vi "Duzy wykres 1.vi"(6 "Wolna?":bool, 8 "error in (no error)":errorcluster, 10 "okno":dbl) -> (0 "error out":errorcluster)   [LabVIEW 2014]
doc: "Use this template to build a VI to use as a subVI."
uses:
  Kontrolki/FVGs/FVG akcje podstawowa.ctl
panel:
  out "Waveform Graph":waveform(dbl)[](graph)
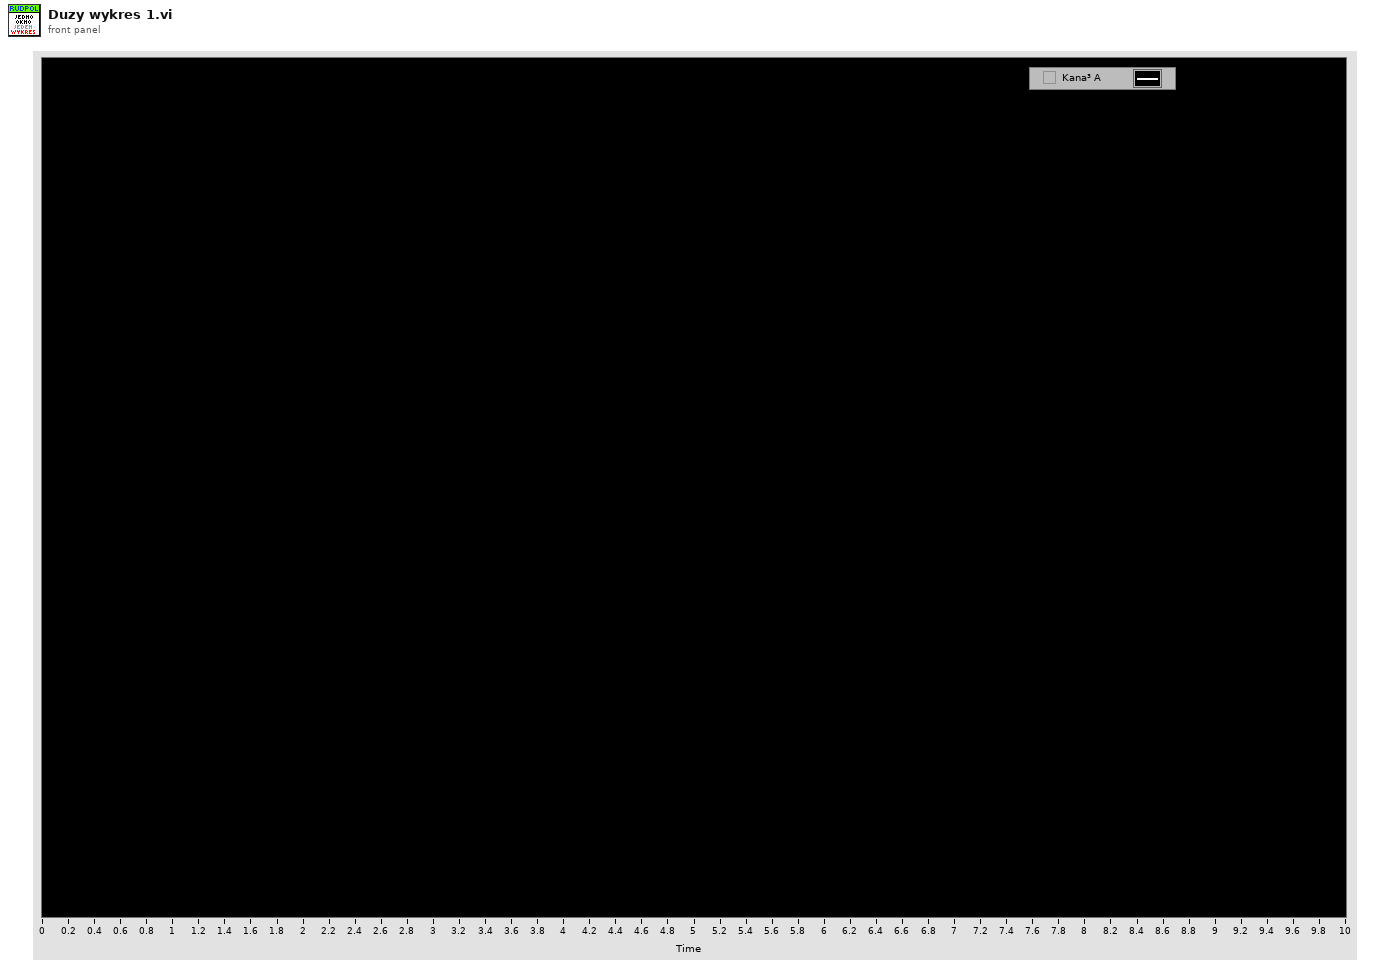
[diagram p1: front panel]
types:
  T1 = typedef "FVG akcje podstawowa.ctl" = enum16{"GET", "SET"}
  T2 = typedef "Kanaly.ctl" = cluster{"Analogowe":waveform(dbl)[], "Cyfrowe":waveform(dbl)[], "Zwarcie":waveform(dbl)[], "Enkoder":waveform(dbl)[]}
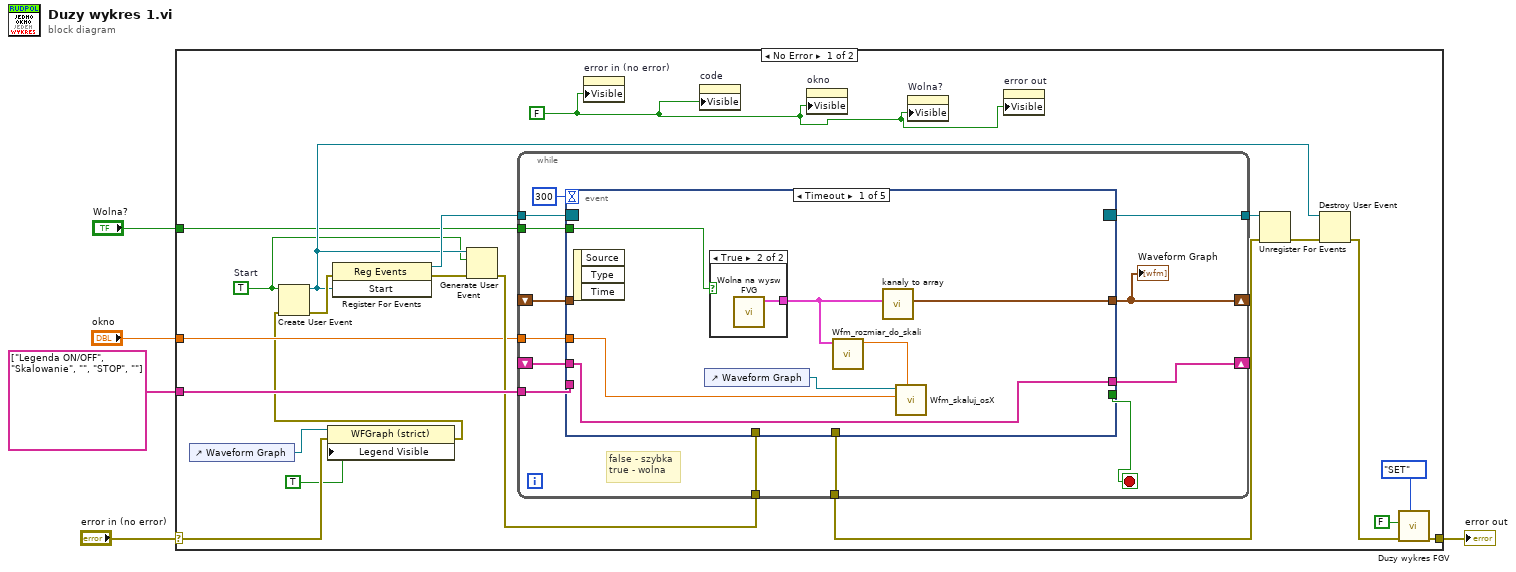
[diagram p0: block diagram]
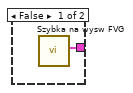
[diagram p2: hidden frame]
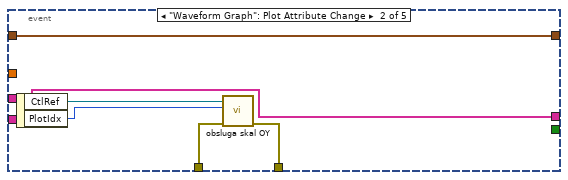
[diagram p3: hidden frame]
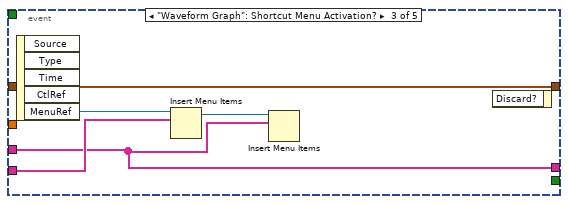
[diagram p4: hidden frame]
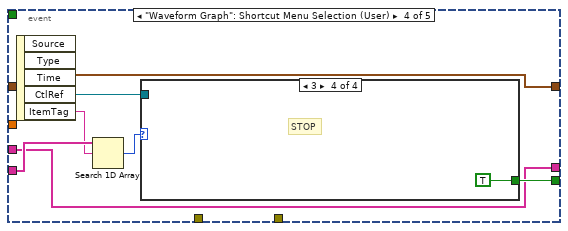
[diagram p5: hidden frame]
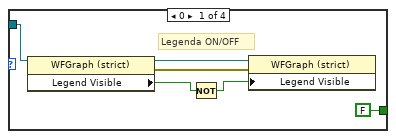
[diagram p6: hidden frame]
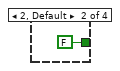
[diagram p7: hidden frame]
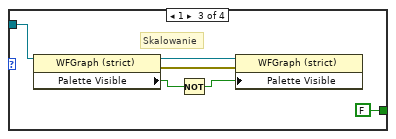
[diagram p8: hidden frame]
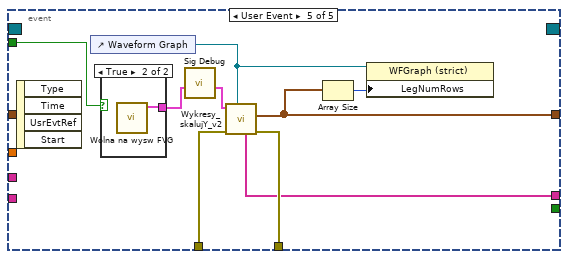
[diagram p9: hidden frame]
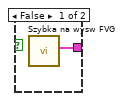
[diagram p10: hidden frame]
diagram:
  n1 = case shown="No Error" "error in (no error)" {
    selector: "error in (no error)" -> [w11 w92]
    tunnel: [w24 w92] -> w4
    tunnel: string[] ["Legenda ON/OFF", "Skalowanie", "", "STOP", ""] -> [w23 _]
    tunnel: "okno" -> [w12 _]
    tunnel: "Wolna?" -> [w7 _]
    frame No Error {
      w13 = TRUE  # Start
      w6 = FALSE ("Visible")
      n2 = control-ref of="Waveform Graph"() -> (w9:refnum<vi>)
      n3 = property class="WFGraph (strict)"(reference=w9, error in=w11, "Legend Visible"=TRUE ("Legend:Visible")) -> (error out=w10:errorcluster)  [unwired: 1 out]
      n4 = Create User Event(user event datatype=w13, error in=w10) -> (user event=w16:refnum<user-event>, error out=w21:errorcluster)
      n5 = register-events(error in=w21, w16) -> (reference out=w22:refnum<event-registration>, error out=w20:errorcluster)  [unwired: 1 in]
      n6 = Generate User Event(user event=w16, event data cluster=w13, error in=w20) -> (error out=w19:errorcluster)  [unwired: 1 in, 1 out]
      n7 = while {
        tunnel: w19 -> [w39]
        tunnel: [w38] -> w15
        tunnel: w23 -> [w36]
        tunnel: w22 -> [w34]
        tunnel: [w33] -> w18
        tunnel: w12 -> [w32]
        shift-right: [w31] -> _
        shift-left: _ -> [w30]
        tunnel: w7 -> [w29]
        shift-right: [w28] -> _
        shift-left: _ -> [w27]
        stop <- w35 stop-if-true
        # "false - szybka\ntrue - wolna"
        n8 = event shown="[0] Timeout" {
          selector: w34 -> [_ _ _ _ _]
          dyn-events: [_ _ _ _ _] -> w33
          timeout: 300 -> [_ _ _ _ _]
          tunnel: w39 -> [_ w51 _ _ w88]
          tunnel: [_ w50 _ _ w87] -> w38
          tunnel: w36 -> [_ _ w58 w66 _]
          tunnel: [_ _ _ w62 _] -> w35
          tunnel: [w46 w52 w57 w61 w86] -> w31
          tunnel: w32 -> [w42 _ _ _ _]
          tunnel: w30 -> [_ w52 w57 w61 _]
          tunnel: w29 -> [w41 _ _ _ w84]
          tunnel: [w40 w49 w56 w60 w81] -> w28
          tunnel: w27 -> [w40 w49 w56 w60 _]
          event Timeout {
            n9 = event-data() -> ()  [unwired: 1 in, 3 out]
            n10 = control-ref of="Waveform Graph"() -> (w43:refnum<vi>)
            n11 = case shown="True" w41 {
              tunnel: [w47 w48] -> w45
              frame False {
                n12 = call "Szybka na wysw FVG.vi"() -> ("Bufor out"=w47:T2)  [unwired: 7 in, 4 out]
              }
              frame True {
                n13 = call "Wolna na wysw FVG.vi"() -> ("Wolna out"=w48:T2)  [unwired: 9 in, 2 out]
              }
            }
            n14 = call "Wfm_rozmiar_do_skali.vi"("Bufor in"=w45) -> ("Size (s)"=w44:dbl)  [unwired: 10 in]
            n15 = call "kanaly to array.vi"("Kanaly"=w45) -> ("Kanaly Array"=w46:waveform(dbl)[])  [unwired: 9 in, 1 out]
            n16 = call "Wfm_skaluj_osX.vi"("size(s)"=w44, "Zakres wysw"=w42, "Waveform in"=w43) -> ()  [unwired: 8 in, 1 out]
          }
          event "Waveform Graph": Plot Attribute Change {
            n17 = event-data() -> ("CtlRef"=w53:refnum<vi>, "PlotIdx"=w54:i32)  [unwired: 1 in]
            n18 = call "obsluga skal OY.vi"("error in (no error)"=w51, "PlotIdx"=w54, "WaveformGraph in"=w53) -> ("error out"=w50:errorcluster)  [unwired: 8 in]
          }
          event "Waveform Graph": Shortcut Menu Activation? {
            n19 = event-data() -> ("MenuRef"=w59:refnum<k9>)  [unwired: 1 in, 4 out]
            n20 = Insert Menu Items(8:w58, 9:w59) -> (3:w55:refnum<k9>)  [unwired: 4 in, 2 out]
            n21 = Insert Menu Items(8:w56, 9:w55) -> ()  [unwired: 4 in, 3 out]
            n22 = event-data() -> ()  [unwired: 2 in, 1 out]
          }
          event "Waveform Graph": Shortcut Menu Selection (User) {
            n23 = event-data() -> ("CtlRef"=w63:refnum<vi>, "ItemTag"=w65:string)  [unwired: 1 in, 3 out]
            n24 = Search 1D Array(1D array=w66, element=w65) -> (index of element=w64:i32)  [unwired: 1 in]
            n25 = case shown="3" w64 {
              tunnel: w63 -> [w68 _ w75 _]
              tunnel: [FALSE FALSE FALSE TRUE] -> w62
              frame 0 {
                # "Legenda ON/OFF"
                n26 = property class="WFGraph (strict)"(reference=w68) -> (reference out=w69:refnum<vi>, error out=w70:errorcluster, "Legend Visible"=w71:bool)  [unwired: 1 in]
                n27 = Not(x=w71) -> (.not. x?=w72:bool)
                n28 = property class="WFGraph (strict)"(reference=w69, error in=w70, "Legend Visible"=w72) -> ()  [unwired: 2 out]
              }
              frame 2, Default {
              }
              frame 1 {
                # "Skalowanie"
                n29 = property class="WFGraph (strict)"(reference=w75) -> (reference out=w76:refnum<vi>, error out=w77:errorcluster, "Palette Visible"=w78:bool)  [unwired: 1 in]
                n30 = Not(x=w78) -> (.not. x?=w79:bool)
                n31 = property class="WFGraph (strict)"(reference=w76, error in=w77, "Palette Visible"=w79) -> ()  [unwired: 2 out]
              }
              frame 3 {
                # "STOP"
              }
            }
          }
          event User Event {
            n32 = event-data() -> ()  [unwired: 1 in, 4 out]
            n33 = control-ref of="Waveform Graph"() -> (w85:refnum<vi>)
            n34 = case shown="True" w84 {
              tunnel: [w90 w91] -> w83
              frame False {
                n35 = call "Szybka na wysw FVG.vi"() -> ("Bufor out"=w90:T2)  [unwired: 7 in, 4 out]
              }
              frame True {
                n36 = call "Wolna na wysw FVG.vi"() -> ("Wolna out"=w91:T2)  [unwired: 9 in, 2 out]
              }
            }
            n37 = call "Sig Debug.vi"("Kanaly in"=w83) -> ("Kanaly out"=w82:T2)  [unwired: 8 in, 2 out]
            n38 = call "Wykresy_skalujY_v2.vi"("Wvm Ref in"=w85, "error in (no error)"=w88, "Data in"=w82) -> ("error out"=w87:errorcluster, "Przebiegi Wfm"=w86:waveform(dbl)[], "Kan i zakr"=w81:string[])  [unwired: 6 in]
            n39 = Array Size(array=w86) -> (size(s)=w89:i32)
            n40 = property class="WFGraph (strict)"(reference=w85, "LegNumRows"=w89) -> ()  [unwired: 1 in, 2 out]
          }
        }
        "Waveform Graph" <- w31
      }
      n41 = property on="error in (no error)" class="Clust (strict)"("Visible"=w6) -> ()  [unwired: 2 in, 2 out]
      n42 = property on="code" class="DigNum (strict)"("Visible"=w6) -> ()  [unwired: 2 in, 2 out]
      n43 = property on="okno" class="DigNum (strict)"("Visible"=w6) -> ()  [unwired: 2 in, 2 out]
      n44 = property on="Wolna?" class="Bool (strict)"("Visible"=w6) -> ()  [unwired: 2 in, 2 out]
      n45 = property on="error out" class="Clust (strict)"("Visible"=w6) -> ()  [unwired: 2 in, 2 out]
      n46 = Unregister For Events(event registration refnum=w18, error in=w15) -> (error out=w17:errorcluster)
      n47 = Destroy User Event(user event=w16, error in=w17) -> (error out=w14:errorcluster)
      n48 = call "Duzy wykres FGV.vi"("Akcja"=FVG_akcje_podstawowa."SET", "error in (no error)"=w14, "Okno1 in"=FALSE) -> ("error out"=w24:errorcluster)  [unwired: 7 in, 1 out]
    }
    frame Error {
    }
  }
  "error out" <- w4
